vi "Send Compl Notif with Error.vi"(7 "Message Priority (Normal)":T2=enum."Normal", 8 "error in (no error)":errorcluster, 9 "Completion Notification Data":T1, 10 "Message Type":refnum<class "Compl Notif with Error Msg.lvclass">, 11 "Message Enqueuer":refnum<class "Message Enqueuer.lvclass">) -> (0 "error out":errorcluster, 3 "Message Enqueuer out":refnum<class "Message Enqueuer.lvclass">)   [LabVIEW 2023, in "Async Methods Actor.lvlib" / "Compl Notif with Error Msg.lvclass"]
doc: "This VI sends the message to an actor."
uses:
  Compl Notif with Error Msg.lvclass
  <vilib>/ActorFramework/Message Enqueuer/Message Enqueuer.lvclass
  <vilib>/ActorFramework/Message Enqueuer/Message Priority.ctl
  C:/Projects/Async Methods Actor/Async Methods Actor/Async Methods Actor Messages/Completion Notification Msg/Completion Notification Msg.lvclass
  C:/Program Files/National Instruments/LabVIEW 2023/vi.lib/ActorFramework/Message/Message.lvclass
  Completion Notification Msg/Completion Notification Data.ctl
  Async Message/Async Message.lvclass
  Completion Notification Msg/Completion Notification Msg.lvclass/Completion Notification Msg.ctl
  <vilib>/ActorFramework/Message Enqueuer/Message Enqueuer.lvclass/Message Enqueuer.ctl
  Completion Notification Msg/Write Async Message.vi
  Completion Notification Msg/Write Current Execution Count.vi
  <vilib>/Utility/LVClass/Get LV Class Name.vi
  <resource>/AFDebug/Generate Trace for Message.vi
  <vilib>/ActorFramework/Message Priority Queue/Priority Enqueue.vi
  <vilib>/ActorFramework/Message/Message.lvclass
  Completion Notification Msg/Completion Notification Msg.lvclass
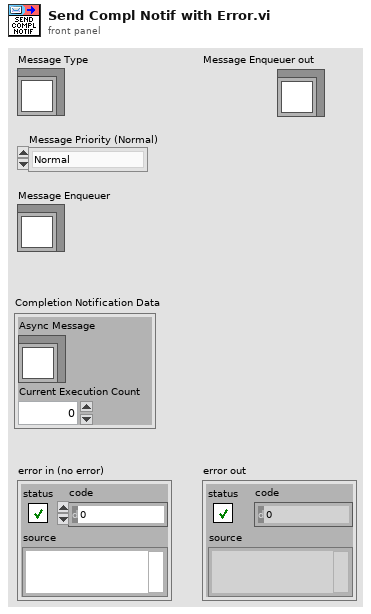
[diagram p1: front panel]
types:
  T1 = typedef "Async Methods Actor.lvlib/Completion Notification Msg.lvclass/Completion Notification Data.ctl" = cluster{"Async Message":refnum<class "Async Message.lvclass">, "Current Execution Count":u32}
  T2 = typedef "Actor Framework.lvlib/Message Enqueuer.lvclass/Message Priority.ctl" = enum16{"Low", "Normal", "High"}
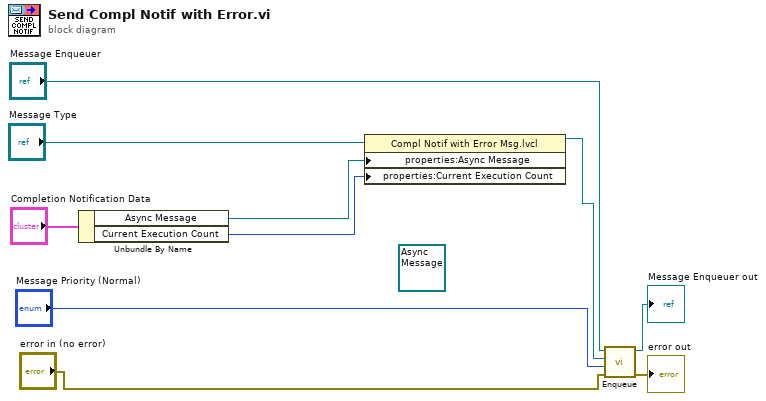
[diagram p0: block diagram]
diagram:
  (unwired) refnum<class "Async Message.lvclass"> refnum ("Async Message")
  n1 = Unbundle By Name("Completion Notification Data") -> ("Async Message"=w1:refnum<class "Async Message.lvclass">, "Current Execution Count"=w2:u32)
  n2 = property class="Compl Notif with Error Msg.lvcl"(reference="Message Type", "properties:Async Message"=w1, "properties:Current Execution Count"=w2) -> (reference out=w3:refnum<class "Compl Notif with Error Msg.lvclass">)  [unwired: 1 in, 1 out]
  n3 = call <vilib>:"Enqueue.vi"("error in (no error)"="error in (no error)", "Message Priority (Normal)"="Message Priority (Normal)", "Message"=w3, "Message Enqueuer in"="Message Enqueuer") -> ("error out"=→"error out":errorcluster, "Message Enqueuer out"=→"Message Enqueuer out":refnum<class "Message Enqueuer.lvclass">)  [unwired: 6 in]
